vi "使用局部变量改变控制控件的值.vi"() -> ()   [LabVIEW 2022 SP3]
doc: "本VI是为《我和LabVIEW》一书编写的示例。\n关于本书的介绍请参考网页：\nhttp://ruanqizhen.spaces.live.com/blog/cns!5852D4F797C53FB6!4310.entry"
panel:
  in  "停止":bool
  in  "字符串":string
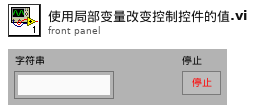
[diagram p1: front panel]
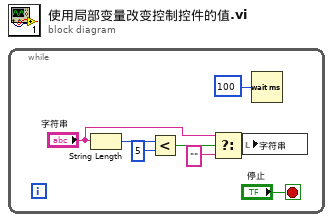
[diagram p0: block diagram]
diagram:
  n1 = while {
    stop <- "停止" stop-if-true
    n2 = String Length(string="字符串") -> (length=w2:i32)
    n3 = Less?(x=w2, y=5) -> (x < y?=w7:bool)
    n4 = Select(t="字符串", s=w7, f="" ("字符串")) -> (s? t:f=w6:string)
    n5 = local write "字符串"(w6) -> ()
    n6 = Wait (ms)(milliseconds to wait=u32 100 ("等待时间（毫秒）")) -> ()  [unwired: 1 out]
  }
